vi "SinglePoint.AddChannels.vi"(8 "Error in":errorcluster, 11 "Waveform Section Refs":T1[](array[typedef]) format="%.0x") -> (0 "Error out":errorcluster)   [LabVIEW 2015, in "SinglePoint.lvlib"]
uses:
  SinglePoint.lvlib
  <vilib>/NI VeriStand/Custom Device API/Custom Device API.lvlib
  Constants.vi
  Waveform-Processing-Custom-Device Shared.lvlib
  <vilib>/NI Veristand/Custom Device API/Get Item Property (Dependent Node Pointer).vi
  <vilib>/NI Veristand/Custom Device API/Custom Device Channel Type.ctl
  <vilib>/NI Veristand/Custom Device API/Custom Device Channel.ctl
  NationalInstruments.VeriStand.SystemStorage
  <vilib>/NI Veristand/Custom Device API/Set Item Property (Dependent Node Pointer).vi
  <vilib>/NI Veristand/Custom Device API/Custom Device Item Ref.ctl
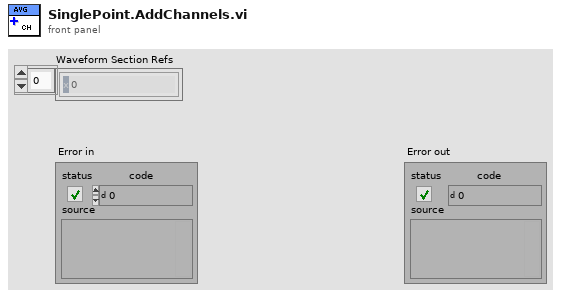
[diagram p1: front panel]
types:
  T1 = typedef "Custom Device API.lvlib/Custom Device Item Ref.ctl" = u64
  T2 = typedef "Custom Device API.lvlib/Custom Device Channel.ctl" = cluster{"Type":T3, "Units":string, "Default Value":dbl, "Faultable":bool, "Scalable":bool}
  T3 = typedef "Custom Device API.lvlib/Custom Device Channel Type.ctl" = enum16{"Input", "Output"}
  T4 = typedef "Custom Device API.lvlib/Custom Device Pointer.ctl" = refnum<k24>
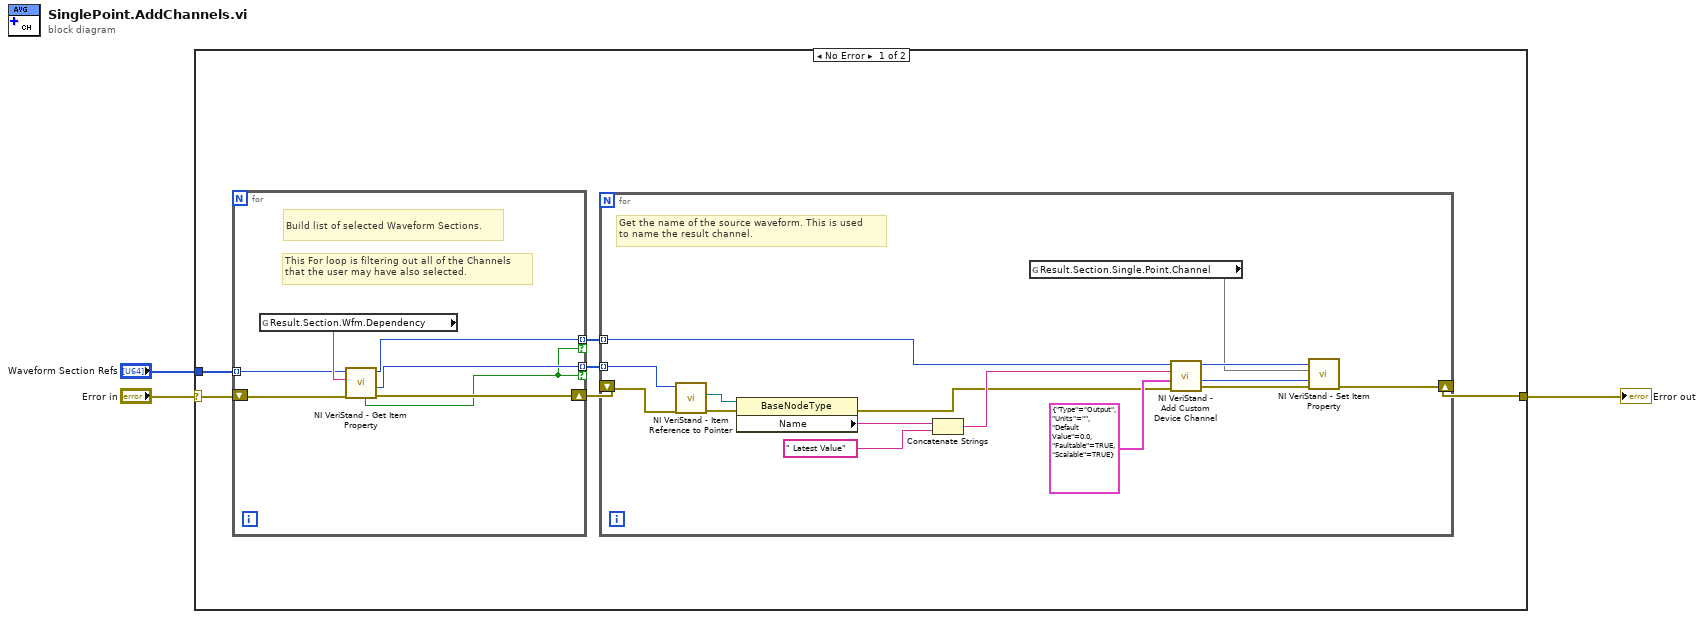
[diagram p0: block diagram]
diagram:
  n1 = case shown="No Error" "Error in" {
    selector: "Error in" -> [w7 w32]
    tunnel: [w9 w32] -> w2
    tunnel: "Waveform Section Refs" -> [w8 _]
    frame No Error {
      n2 = for {
        tunnel: w8 -> [w15] mode=indexing
        shift-right: [w13] -> w6
        shift-left: w7 -> [w14]
        tunnel: [w12] -> w5 mode=indexing if=w10
        tunnel: [w11] -> w4 mode=indexing if=w10
        # "This For loop is filtering out all of the Channels\nthat the user may have also selected."
        # "Build list of selected Waveform Sections."
        n3 = global read "Constants.vi" "Result.Section.Wfm.Dependency"() -> (w16:string)
        n4 = call-poly <vilib>:"NI VeriStand - Get Item Property.vi"("error in (no error)"=w14, "Property Name"=w16, "Item Ref in"=w15) -> ("error out"=w13:errorcluster, "Dependent Node Ref"=w12:T1, "Item Ref out"=w11:T1, "Found"=w10:bool)  [unwired: 5 in]
      }
      n5 = for {
        shift-right: [w20] -> w9
        shift-left: w6 -> [w19]
        tunnel: w5 -> [w18] mode=indexing
        tunnel: w4 -> [w17] mode=indexing
        # "Get the name of the source waveform. This is used\nto name the result channel."
        n6 = call <vilib>:"NI VeriStand - Item Reference to Pointer.vi"("error in (no error)"=w19, "Item Ref in"=w18) -> ("error out"=w29:errorcluster, "Node Pointer"=w25:T4)  [unwired: 6 in, 2 out]
        n7 = property class="BaseNodeType"(reference=w25, error in=w29) -> (error out=w26:errorcluster, "Name"=w28:string)  [unwired: 1 out]
        n8 = Concatenate Strings(w28, " Latest Value" ("Property Name")) -> (w31:string)
        n9 = global read "Constants.vi" "Result.Section.Single.Point.Channel"() -> (w22)
        n10 = call <vilib>:"NI VeriStand - Add Custom Device Channel.vi"("error in (no error)"=w26, "Channel"=T2 {"Type"=enum."Output", "Units"="", "Default Value"=0.0, "Faultable"=TRUE, "Scalable"=TRUE}, "Channel Name"=w31, "Parent Ref in"=w17) -> ("error out"=w21:errorcluster, "Channel Ref"=w23:T1, "Parent Ref out"=w24:T1)  [unwired: 4 in, 1 out]
        n11 = call-poly <vilib>:"NI VeriStand - Set Item Property.vi"("error in (no error)"=w21, "Dependent Node Ref"=w23, "Property Name"=w22, "Item Ref in"=w24) -> ("error out"=w20:errorcluster)  [unwired: 5 in, 2 out]
      }
    }
    frame Error {
    }
  }
  "Error out" <- w2
